vi "Control - PFI - Cranking.vi"(0 "Control Inputs":T4={"Engine Speed [RPM]"=0.0, "Engine Status"=enum."STALLED", "Load Control \nMode"=enum."High-Idle Governor", "dt(s)"=0.0, "Number of Cylinders"=0, "Engine Displacement [cc]"=0.0, "StoichAFR"=0.0, "Q.LHV Fuel [kJ/kg]"=0.0, "BattV PSU [V]"=0.0, "12V PSU [V]"=0.0, "5V PSU [V]"=0.0, "Pedal Position [%]"=0.0, "Oil Pressure [kPa]"=0.0, "Oil Temp [C]"=0.0, "Oil Level [%]"=0.0, "Engine Coolant Temp (ECT) [C]"=0.0, "Engine Coolant Pressure [kPa]"=0.0, "Rail Pressure [bar]"=0.0, "Fuel Pressure [kPa]"=0.0, "Fuel Temp [C]"=0.0, "Vacuum Pressure [kPa]"=0.0, "Throttle Position [%]"=0.0, "Cam1 Advance [CAD]"=0.0, "Cam2 Advance [CAD]"=0.0, "Cam3 Advance [CAD]"=0.0, "Cam4 Advance [CAD]"=0.0, "CA50 Control Output [CAD]"=[], "CA50 Control Output Valid"=[], "Intake Air Temp (IAT) [C]"=0.0, "Barometric Air Pressure [kPa]"=0.0, "Intake Air Rel. Humidity [%]"=0.0, "Mass Air Flow (MAF) [kg/hr]"=0.0, "Turbo Inlet Air Pressure [kPa]"=0.0, "Turbo Inlet Air Temp [C]"=0.0, "Turbo Outlet Air Pressure [kPa]"=0.0, "Turbo Outlet Air Temp [C]"=0.0, "CAC Outlet Pressure [kPa]"=0.0, "CAC Outlet Temp [C]"=0.0, "Intake Manifold Pressure (MAP) [kPa]"=0.0, "Intake Manifold Temp (MAT) [C]"=0.0, "Exhaust Manifold Pressure [kPa]"=0.0, "Exhaust Manifold Temp [C]"=0.0, "HighP EGR Cooler Outlet Pressure [kPa]"=0.0, "HighP EGR Cooler Outlet Temp [C]"=0.0, "HighP EGR Differential Pressure [kPa]"=0.0, "HighP EGR Valve Position [%]"=0.0, "Turbo Outlet Exhaust Pressure [kPa]"=0.0, "Turbo Outlet Exhaust Temp [C]"=0.0, "VGT Position 1 [%]"=0.0, "VGT Position 2 [%]"=0.0, "Turbo Speed 1 [RPM]"=0.0, "Turbo Speed 2 [RPM]"=0.0, "LowP EGR Differential Pressure [kPa]"=0.0, "LowP EGR Valve Position [%]"=0.0, "UEGO1Lambda"=0.0, "UEGO1_Hot"=FALSE, "UEGO2Lambda"=0.0, "UEGO2_Hot"=FALSE, "Knock Intensity"=[], "Knock"=[]} {"Knock Intensity" format="%.2f"; "CA50 Control Output [CAD]" format="%.2f"; "Exhaust Manifold Temp [C]" format="%#_6f"; "UEGO2Lambda" format="%.2f"; "Intake Manifold Temp (MAT) [C]" format="%#_6f"; "UEGO1Lambda" format="%.2f"}, 1 "Available Air Mass [mg/cyc]":sgl, 5 "Control Outputs In":T1) -> (19 "Control Outputs":T1)   [LabVIEW 2015, in "ECS-RT.lvlib"]
uses:
  ECS-RT.lvlib
  Typedefs/Control Inputs/Control Inputs.ctl
  Typedefs/EPT/Engine Status.ctl
  Typedefs/MISC/Load Control Mode.ctl
  Typedefs/Control Outputs/Control Outputs.ctl
  Typedefs/Control Outputs/Injection Quantity.ctl
  Typedefs/Control Outputs/Injection Timing.ctl
  ECS-Shared.lvlib
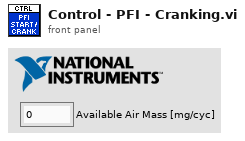
[diagram p1: front panel]
types:
  T1 = typedef "ECS-Shared.lvlib/Control Outputs.ctl" = cluster{"Pedal Desired [%]":sgl, "MEP Desired [bar]":sgl, "Fuel Desired [mg/cyc]":sgl, "Intake MAP Desired [kPa]":sgl, "Cam1 Advance Setpoint [CAD]":sgl, "Cam2 Advance Setpoint [CAD]":sgl, "HighP EGR Position Setpoint [%Open]":sgl, "LowP EGR Position Setpoint [%Open]":sgl, "Rail Pressure Setpoint [bar]":sgl, "Wastegate1 Position Setpoint [%Open]":sgl, "Wastegate2 Position Setpoint [%Open]":sgl, "VGT1 Position Setpoint [%Open]":sgl, "VGT2 Position Setpoint [%Open]":sgl, "Throttle1 Position Setpoint [%Open]":sgl, "Throttle2 Position Setpoint [%Open]":sgl, "TurboBPV Position Setpoint [%Open]":sgl, "Spark Dwells [msec]":sgl[], "Spark Timings [DBTDC]":sgl[], "PFI Quantities [mg/inj]":sgl[], "PFI Timings [DBTDC]":sgl[], "DI Quantities [mg/inj]":T2[], "DI Timings [DBTDC]":T3[]}
  T2 = typedef "ECS-Shared.lvlib/Injection Quantity.ctl" = cluster{"Pilot1Quantity [mg/inj]":sgl, "Pilot2Quantity [mg/inj]":sgl, "MainQuantity [mg/inj]":sgl, "Post1Quantity [mg/inj]":sgl, "Post2Quantity [mg/inj]":sgl}
  T3 = typedef "ECS-Shared.lvlib/Injection Timing.ctl" = cluster{"Pilot1SOI [DBTDC]":sgl, "Pilot2SOI [DBTDC]":sgl, "MainSOI [DBTDC]":sgl, "Post1SOI [DBTDC]":sgl, "Post2SOI [DBTDC]":sgl}
  T4 = typedef "ECS-Shared.lvlib/Control Inputs.ctl" = cluster{"Engine Speed [RPM]":sgl, "Engine Status":T5, "Load Control \nMode":T6, "dt(s)":sgl, "Number of Cylinders":u8, "Engine Displacement [cc]":sgl, "StoichAFR":sgl, "Q.LHV Fuel [kJ/kg]":sgl, "BattV PSU [V]":sgl, "12V PSU [V]":sgl, "5V PSU [V]":sgl, "Pedal Position [%]":sgl, "Oil Pressure [kPa]":sgl, "Oil Temp [C]":sgl, "Oil Level [%]":sgl, "Engine Coolant Temp (ECT) [C]":sgl, "Engine Coolant Pressure [kPa]":sgl, "Rail Pressure [bar]":sgl, "Fuel Pressure [kPa]":sgl, "Fuel Temp [C]":sgl, "Vacuum Pressure [kPa]":sgl, "Throttle Position [%]":sgl, "Cam1 Advance [CAD]":sgl, "Cam2 Advance [CAD]":sgl, "Cam3 Advance [CAD]":sgl, "Cam4 Advance [CAD]":sgl, "CA50 Control Output [CAD]":sgl[], "CA50 Control Output Valid":bool[], "Intake Air Temp (IAT) [C]":sgl, "Barometric Air Pressure [kPa]":sgl, "Intake Air Rel. Humidity [%]":sgl, "Mass Air Flow (MAF) [kg/hr]":sgl, "Turbo Inlet Air Pressure [kPa]":sgl, "Turbo Inlet Air Temp [C]":sgl, "Turbo Outlet Air Pressure [kPa]":sgl, "Turbo Outlet Air Temp [C]":sgl, "CAC Outlet Pressure [kPa]":sgl, "CAC Outlet Temp [C]":sgl, "Intake Manifold Pressure (MAP) [kPa]":sgl, "Intake Manifold Temp (MAT) [C]":sgl, "Exhaust Manifold Pressure [kPa]":sgl, "Exhaust Manifold Temp [C]":sgl, "HighP EGR Cooler Outlet Pressure [kPa]":sgl, "HighP EGR Cooler Outlet Temp [C]":sgl, "HighP EGR Differential Pressure [kPa]":sgl, "HighP EGR Valve Position [%]":sgl, "Turbo Outlet Exhaust Pressure [kPa]":sgl, "Turbo Outlet Exhaust Temp [C]":sgl, "VGT Position 1 [%]":sgl, "VGT Position 2 [%]":sgl, "Turbo Speed 1 [RPM]":sgl, "Turbo Speed 2 [RPM]":sgl, "LowP EGR Differential Pressure [kPa]":sgl, "LowP EGR Valve Position [%]":sgl, "UEGO1Lambda":sgl, "UEGO1_Hot":bool, "UEGO2Lambda":sgl, "UEGO2_Hot":bool, "Knock Intensity":sgl[], "Knock":bool[]}
  T5 = typedef "ECS-Shared.lvlib/Engine Status.ctl" = enum16{"OFF", "STALLED", "CRANKING", "RUNNING", "ACCEL", "DECEL", "SAFE"}
  T6 = typedef "ECS-Shared.lvlib/Load Control Mode.ctl" = enum16{"No Governor", "Low-Idle Governor", "High-Idle Governor"}
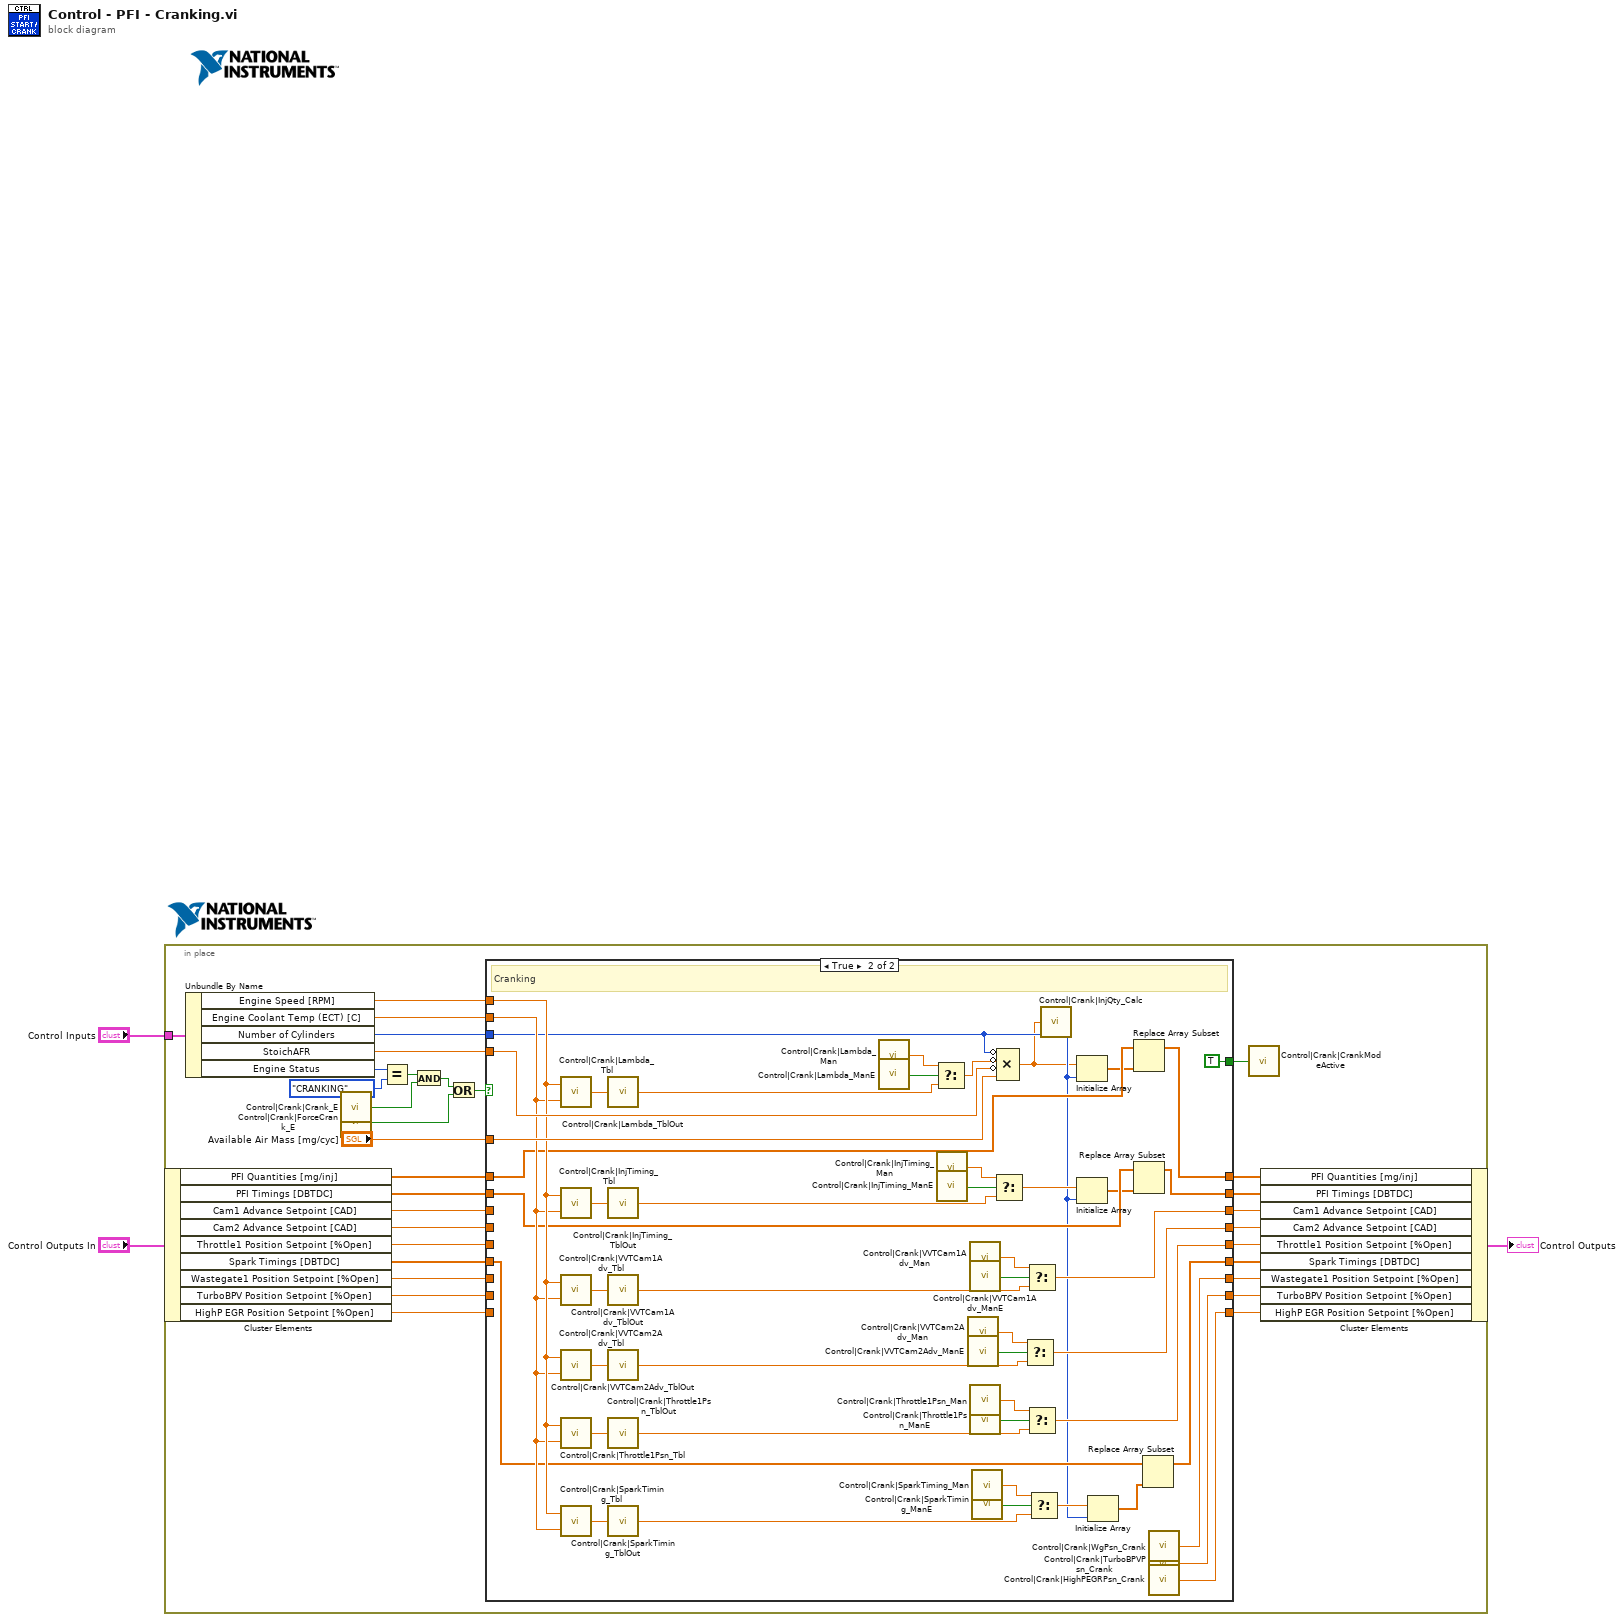
[diagram p0: block diagram]
diagram:
  n1 = in-place {
    in-place-border: "Control Inputs" -> [w31]
    n2 = in-place-cluster #1("Control Outputs In") -> ("PFI Quantities [mg/inj]"=w5:sgl[], "PFI Timings [DBTDC]"=w4:sgl[], "Cam1 Advance Setpoint [CAD]"=w16:sgl, "Cam2 Advance Setpoint [CAD]"=w17:sgl, "Throttle1 Position Setpoint [%Open]"=w18:sgl, "Spark Timings [DBTDC]"=w7:sgl[], "Wastegate1 Position Setpoint [%Open]"=w19:sgl, "TurboBPV Position Setpoint [%Open]"=w20:sgl, "HighP EGR Position Setpoint [%Open]"=w21:sgl)
    n3 = Unbundle By Name(w31) -> ("Engine Speed [RPM]"=w35:sgl, "Engine Coolant Temp (ECT) [C]"=w34:sgl, "Number of Cylinders"=w33:u8, "StoichAFR"=w32:sgl, "Engine Status"=w29:T5)
    n4 = call "Control|Crank|Crank_E"() -> ("Value"=w26:bool)
    n5 = call "Control|Crank|ForceCrank_E"() -> ("Value"=w24:bool)
    n6 = Equal?(x=w29, y=Engine_Status."CRANKING" ("Engine Status")) -> (x = y?=w27:bool)
    n7 = And(x=w27, y=w26) -> (x .and. y?=w23:bool)
    n8 = Or(x=w23, y=w24) -> (x .or. y?=w25:bool)
    n9 = case shown="True" w25 {
      tunnel: w35 -> [_ w59]
      tunnel: w34 -> [_ w58]
      tunnel: w33 -> [_ w46]
      tunnel: w32 -> [_ w70]
      tunnel: "Available Air Mass [mg/cyc]" -> [_ w69]
      tunnel: [_ TRUE] -> w30
      tunnel: w21 -> [w37 _]
      tunnel: w20 -> [w38 _]
      tunnel: w19 -> [w39 _]
      tunnel: w18 -> [w40 _]
      tunnel: w17 -> [w41 _]
      tunnel: w16 -> [w42 _]
      tunnel: w4 -> [w43 w53]
      tunnel: w5 -> [w44 w52]
      tunnel: [w44 w51] -> w15
      tunnel: [w43 w50] -> w14
      tunnel: [w42 w62] -> w13
      tunnel: [w41 w61] -> w12
      tunnel: [w40 w60] -> w11
      tunnel: [w39 w75] -> w10
      tunnel: [w38 w76] -> w9
      tunnel: [w37 w77] -> w8
      tunnel: w7 -> [w36 w57]
      tunnel: [w36 w54] -> w6
      frame False {
        # "Normal Operation"
      }
      frame True {
        # "Cranking"
        n10 = call "Control|Crank|Lambda_Tbl"("Y Index"=w58, "X Index"=w59) -> ("Z"=w72:sgl)
        n11 = call "Control|Crank|InjTiming_Tbl"("Y Index"=w58, "X Index"=w59) -> ("Z"=w68:sgl)
        n12 = call "Control|Crank|VVTCam1Adv_Tbl"("Y Index"=w58, "X Index"=w59) -> ("Z"=w63:sgl)
        n13 = call "Control|Crank|VVTCam2Adv_Tbl"("Y Index"=w58, "X Index"=w59) -> ("Z"=w83:sgl)
        n14 = call "Control|Crank|Throttle1Psn_Tbl"("Y Index"=w58, "X Index"=w59) -> ("Z"=w84:sgl)
        n15 = call "Control|Crank|SparkTiming_Tbl"("Y Index"=w58, "X Index"=w59) -> ("Z"=w80:sgl)
        n16 = call "Control|Crank|Lambda_TblOut"("Value"=w72) -> ()
        n17 = call "Control|Crank|InjTiming_TblOut"("Value"=w68) -> ()
        n18 = call "Control|Crank|VVTCam1Adv_TblOut"("Value"=w63) -> ()
        n19 = call "Control|Crank|VVTCam2Adv_TblOut"("Value"=w83) -> ()
        n20 = call "Control|Crank|Throttle1Psn_TblOut"("Value"=w84) -> ()
        n21 = call "Control|Crank|SparkTiming_TblOut"("Value"=w80) -> ()
        n22 = call "Control|Crank|Lambda_Man"() -> ("Value"=w74:sgl)
        n23 = call "Control|Crank|Lambda_ManE"() -> ("Value"=w73:bool)
        n24 = Select(t=w74, s=w73, f=w72) -> (s? t:f=w71:sgl)
        n25 = call "Control|Crank|InjTiming_Man"() -> ("Value"=w67:sgl)
        n26 = call "Control|Crank|InjTiming_ManE"() -> ("Value"=w66:bool)
        n27 = call "Control|Crank|VVTCam2Adv_Man"() -> ("Value"=w81:sgl)
        n28 = call "Control|Crank|VVTCam2Adv_ManE"() -> ("Value"=w82:bool)
        n29 = call "Control|Crank|VVTCam1Adv_Man"() -> ("Value"=w65:sgl)
        n30 = call "Control|Crank|VVTCam1Adv_ManE"() -> ("Value"=w64:bool)
        n31 = call "Control|Crank|Throttle1Psn_Man"() -> ("Value"=w86:sgl)
        n32 = call "Control|Crank|Throttle1Psn_ManE"() -> ("Value"=w85:bool)
        n33 = call "Control|Crank|SparkTiming_Man"() -> ("Value"=w79:sgl)
        n34 = call "Control|Crank|SparkTiming_ManE"() -> ("Value"=w78:bool)
        n35 = Select(t=w67, s=w66, f=w68) -> (s? t:f=w49:sgl)
        n36 = Compound Arithmetic op=MULTIPLY(invert w46, invert w71, invert w70, w69) -> (w45:dbl)
        n37 = Select(t=w81, s=w82, f=w83) -> (s? t:f=w61:sgl)
        n38 = Select(t=w65, s=w64, f=w63) -> (s? t:f=w62:sgl)
        n39 = Select(t=w86, s=w85, f=w84) -> (s? t:f=w60:sgl)
        n40 = Select(t=w79, s=w78, f=w80) -> (s? t:f=w56:sgl)
        n41 = call "Control|Crank|InjQty_Calc"("Value"=w45) -> ()
        n42 = Initialize Array(w45, w46) -> (w48:dbl[])
        n43 = Initialize Array(w49, w46) -> (w47:sgl[])
        n44 = Initialize Array(w56, w46) -> (w55:sgl[])
        n45 = Replace Array Subset(array=w52, new element=w48) -> (w51:sgl[])  [unwired: 1 in]
        n46 = Replace Array Subset(array=w53, new element=w47) -> (w50:sgl[])  [unwired: 1 in]
        n47 = Replace Array Subset(array=w57, new element=w55) -> (w54:sgl[])  [unwired: 1 in]
        n48 = call "Control|Crank|WgPsn_Crank"() -> ("Value"=w75:sgl)
        n49 = call "Control|Crank|TurboBPVPsn_Crank"() -> ("Value"=w76:sgl)
        n50 = call "Control|Crank|HighPEGRPsn_Crank"() -> ("Value"=w77:sgl)
      }
    }
    n51 = call "Control|Crank|CrankModeActive"("Value"=w30) -> ()
    n52 = in-place-cluster #1("PFI Quantities [mg/inj]"=w15, "PFI Timings [DBTDC]"=w14, "Cam1 Advance Setpoint [CAD]"=w13, "Cam2 Advance Setpoint [CAD]"=w12, "Throttle1 Position Setpoint [%Open]"=w11, "Spark Timings [DBTDC]"=w6, "Wastegate1 Position Setpoint [%Open]"=w10, "TurboBPV Position Setpoint [%Open]"=w9, "HighP EGR Position Setpoint [%Open]"=w8) -> (→"Control Outputs":T1)
  }
